vi "Drive Forward Drive.vi"(8 "error in (no error)":errorcluster, 10 "Joystick State":T1, 11 "Driver in":refnum<class "Driver.lvclass">) -> (0 "error out":errorcluster, 3 "Driver out":refnum<class "Driver.lvclass">)   [LabVIEW 2014, in "Driver.lvlib" / "Driver.lvclass"]
uses:
  Driver.lvclass
  Joystick/Joystick Class/Joystick State.ctl
  Joystick/Joystick Class/Button State.ctl
  Joystick/Joystick Class/Axis State.ctl
  Driver.lvclass/Driver.ctl
  Forward Drive/Forward Drive Messages/Set Percentage Msg/Set Percentage Msg.lvclass/Set Percentage Msg.ctl
  <vilib>/ActorFramework/Message Enqueuer/Message Enqueuer.lvclass/Message Enqueuer.ctl
  <vilib>/ActorFramework/Message Enqueuer/Enqueue.vi
  <vilib>/ActorFramework/Message Priority Queue/Priority Enqueue.vi
  Forward Drive/Forward Drive Messages/Set Percentage Msg/Set Percentage Msg.lvclass
  Joystick/Joystick.lvlib
  Joystick/Joystick Class/Joystick.lvclass
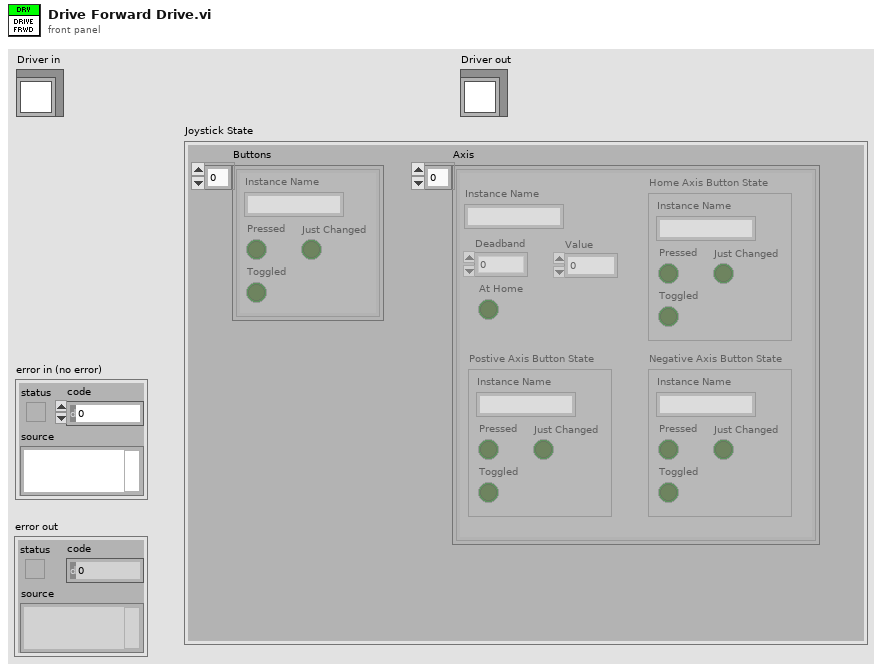
[diagram p1: front panel]
types:
  T1 = typedef "Joystick.lvlib/Joystick.lvclass/Joystick State.ctl" = cluster{"Buttons":T2[], "Axis":T3[]}
  T2 = typedef "Joystick.lvlib/Joystick.lvclass/Button State.ctl" = cluster{"Pressed":bool, "Instance Name":string, "Toggled":bool, "Just Changed":bool}
  T3 = typedef "Joystick.lvlib/Joystick.lvclass/Axis State.ctl" = cluster{"Instance Name":string, "Deadband":dbl, "Value":dbl, "At Home":bool, "Postive Axis Button State":T2, "Negative Axis Button State":T2, "Home Axis Button State":T2}
  T4 = enum16{"Critical", "Error", "Warning", "Informational", "Debug"}
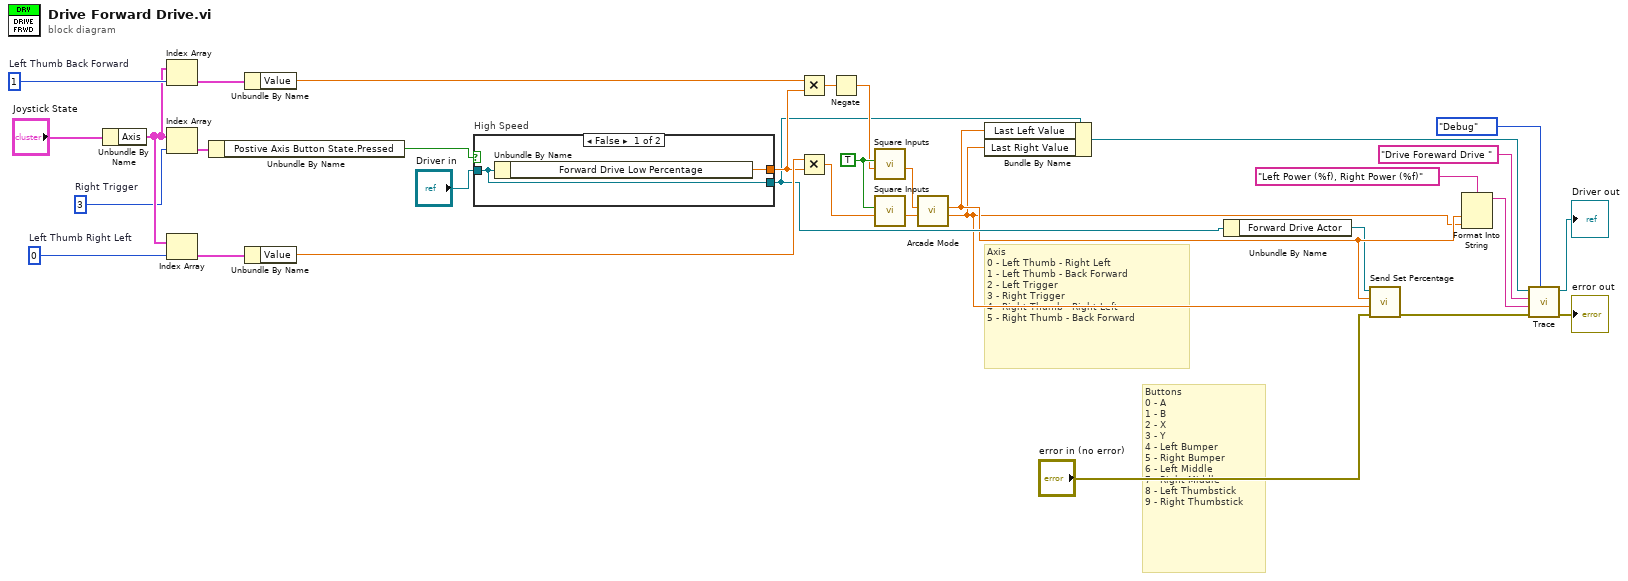
[diagram p0: block diagram]
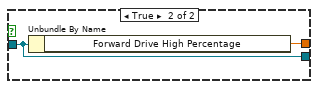
[diagram p2: hidden frame]
diagram:
  w12 = 3  # Right Trigger
  w22 = 0  # Left Thumb Right Left
  w23 = 1  # Left Thumb Back Forward
  w30 = TRUE ("Square Inputs")
  # "Buttons\n0 - A\n1 - B\n2 - X\n3 - Y\n4 - Left Bumper\n5 - Right Bumper\n6 - Left Middle\n7 - Right Middle\n8 - Left Thumbstick\n9 - Right Thumbstick"
  # "Axis\n0 - Left Thumb - Right Left\n1 - Left Thumb - Back Forward\n2 - Left Trigger\n3 - Right Trigger\n4 - Right Thumb - Right Left\n5 - Right Thumb - Back Forward"
  n1 = Unbundle By Name("Joystick State") -> ("Axis"=w13:T3[])
  n2 = Index Array(array=w13, index=w23) -> (element=w19:T3)
  n3 = Index Array(array=w13, index=w12) -> (element=w11:T3)
  n4 = Index Array(array=w13, index=w22) -> (element=w21:T3)
  n5 = Unbundle By Name(w11) -> ("Postive Axis Button State.Pressed"=w10:bool)
  n6 = Unbundle By Name(w19) -> ("Value"=w18:dbl)
  n7 = Unbundle By Name(w21) -> ("Value"=w20:dbl)
  n8 = case "High Speed" shown="False" w10 {
    tunnel: "Driver in" -> [w34 w36]
    tunnel: [w34 w36] -> w5
    tunnel: [w33 w35] -> w8
    frame False {
      n9 = Unbundle By Name(w34) -> ("Forward Drive Low Percentage"=w33:dbl)
    }
    frame True {
      n10 = Unbundle By Name(w36) -> ("Forward Drive High Percentage"=w35:dbl)
    }
  }
  n11 = Multiply(x=w18, y=w8) -> (x*y=w15:dbl)
  n12 = Multiply(x=w20, y=w8) -> (x*y=w14:dbl)
  n13 = Negate(x=w15) -> (-x=w24:dbl)
  n14 = call "Square Inputs.vi"("Before Square"=w24, "Square Inputs"=w30) -> ("After Square"=w29:dbl)  [unwired: 9 in]
  n15 = call "Square Inputs.vi"("Before Square"=w14, "Square Inputs"=w30) -> ("After Square"=w28:dbl)  [unwired: 9 in]
  n16 = call "Arcade Mode.vi"("Right Joystick"=w28, "Forward Joystick"=w29) -> ("Right Power"=w3:dbl, "Left Power"=w4:dbl)  [unwired: 8 in]
  n17 = Bundle By Name(cluster=w5, "Last Left Value"=w4, "Last Right Value"=w3) -> (w2:refnum<class "Driver.lvclass">)
  n18 = Unbundle By Name(w5) -> ("Forward Drive Actor"=w1:refnum<class "Message Enqueuer.lvclass">)
  n19 = call "Send Set Percentage.vi"("error in (no error)"="error in (no error)", "Right Percentage"=w3, "Left Percentage"=w4, "Message Enqueuer"=w1) -> ("error out"=w17:errorcluster)  [unwired: 6 in, 1 out]
  n20 = Format Into String(format string="Left Power (%f), Right Power (%f)", w4, w3) -> (resulting string=w7:string)  [unwired: 2 in, 1 out]
  n21 = call-dynamic "Trace.vi"("Trace Level"=T4."Debug", "error in (no error)"=w17, "System Message"=w7, "System Action"="Drive Foreward Drive ", "System Actor in"=w2) -> ("error out"=→"error out":errorcluster, "System Actor out"=→"Driver out":refnum<class "Driver.lvclass">)  [unwired: 5 in]
